vi "Sgl_ReadWriteAttribute.vi"(5 "error in (no error)":errorcluster) -> (19 "error out":errorcluster)   [LabVIEW 2012, in "SingletonTemplate.lvclass"]
uses:
  <resource>/Framework/Providers/Open_GDS/ClassProviders/Provider_EndevoGOOP300/Templates/SingletonTemplate/SingletonTemplate.lvclass
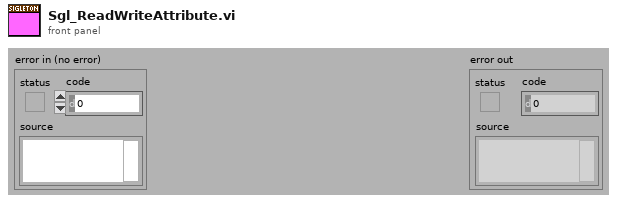
[diagram p1: front panel]
types:
  T1 = typedef "SingletonTemplate.lvclass/ObjectAttributes.ctl" = cluster{"Attribute1":dbl}
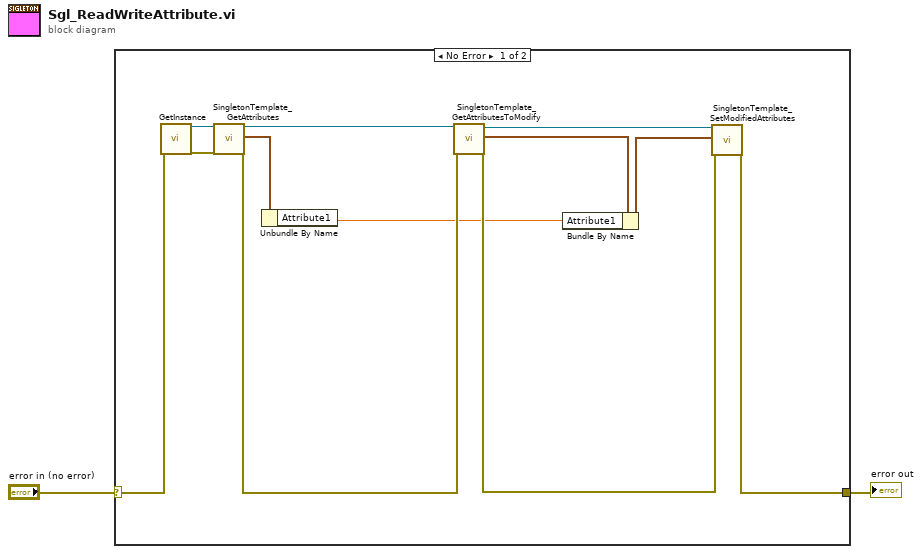
[diagram p0: block diagram]
diagram:
  n1 = case shown="No Error" "error in (no error)" {
    selector: "error in (no error)" -> [w4 w15]
    tunnel: [w11 w15] -> w1
    frame No Error {
      n2 = call <resource>:"GetInstance.vi"("error in (no error)"=w4) -> ("reference out"=w3:refnum<class "SingletonTemplate.lvclass">, "error out"=w5:errorcluster)  [unwired: 17 in]
      n3 = call <resource>:"SingletonTemplate_GetAttributes.vi"("reference in"=w3, "error in (no error)"=w5) -> ("reference out"=w8:refnum<class "SingletonTemplate.lvclass">, "Attributes"=w7:T1, "error out"=w9:errorcluster)  [unwired: 14 in, 1 out]
      n4 = Unbundle By Name(w7) -> ("Attribute1"=w6:dbl)
      n5 = call <resource>:"SingletonTemplate_GetAttributesToModify.vi"("reference in"=w8, "error in (no error)"=w9) -> ("reference out"=w12:refnum<class "SingletonTemplate.lvclass">, "Attributes"=w14:T1, "error out"=w10:errorcluster)  [unwired: 14 in, 1 out]
      n6 = Bundle By Name(cluster=w14, "Attribute1"=w6) -> (w13:T1)
      n7 = call <resource>:"SingletonTemplate_SetModifiedAttributes.vi"("reference in"=w12, "Attributes"=w13, "error in (no error)"=w10) -> ("error out"=w11:errorcluster)  [unwired: 15 in, 1 out]
    }
    frame Error {
    }
  }
  "error out" <- w1
